vi "fo_DumpDataset.vi"(8 "error in (no error)":errorcluster, 11 "file":string) -> (0 "error out":errorcluster, 1 "items":string[](array[string]), 2 "keywords":string[](array[string]), 3 "tags":string[](array[string]))   [LabVIEW 2013, in "main.lvlib"]
uses:
  main.lvlib
  C:/Users/Simon/SkyDrive/LabView/2013/DM2020/bin/Dicom.dll
  bin/Dicom.dll
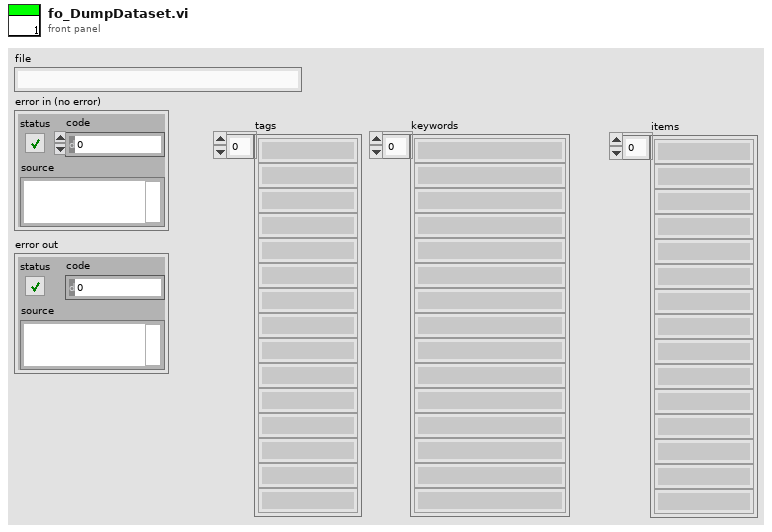
[diagram p1: front panel]
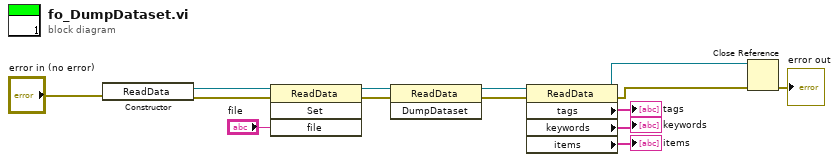
[diagram p0: block diagram]
diagram:
  n1 = constructor class="ReadData"(error in="error in (no error)") -> (reference out=w14:refnum<k24>, error out=w12:errorcluster)  [unwired: 2 in, 1 out]
  n2 = invoke class="ReadData" method="Set"(reference=w14, error in=w12, "file"="file") -> (reference out=w3:refnum<k24>, error out=w4:errorcluster)  [unwired: 1 in, 2 out]
  n3 = invoke class="ReadData" method="DumpDataset"(reference=w3, error in=w4) -> (reference out=w2:refnum<k24>, error out=w1:errorcluster)  [unwired: 1 in, 1 out]
  n4 = property class="ReadData"(reference=w2, error in=w1) -> (reference out=w5:refnum<k24>, error out=w6:errorcluster, "tags"=→"tags":string[], "keywords"=→"keywords":string[], "items"=→"items":string[])
  n5 = Close Reference(reference=w5, error in (no error)=w6) -> (error out=→"error out":errorcluster)
